vi "Intake Get.vi"(6 "Operator Intake In":T3, 8 "Gripper":bool, 9 "Gripper In":bool, 10 "error in (no error)":errorcluster, 11 "Arm State":bool) -> (0 "error out":errorcluster, 1 "Operator Intake Out":T3)   [LabVIEW 2013]
uses:
  <vilib>/Rock Robotics/WPI/Relay/WPI_RelayValue.ctl
  <vilib>/Rock Robotics/WPI/Solenoid/WPI_SolenoidValue.ctl
panel:
  # "0 < Gripper - Intake\n0 = Gripper - stop\n0 > Gripper - Eject"
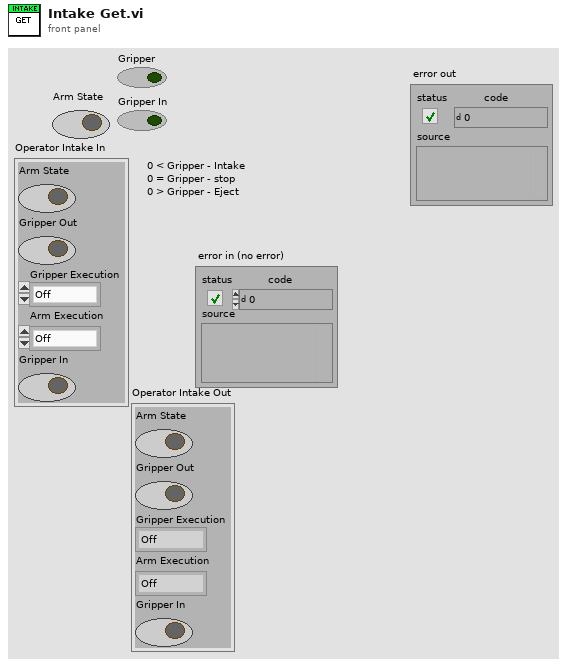
[diagram p1: front panel]
types:
  T1 = typedef "WPI_RelayValue.ctl" = enum16{"Off", "On", "Forward", "Reverse"}
  T2 = typedef "WPI_SolenoidValue.ctl" = enum16{"Off", "On", "Forward", "Reverse"}
  T3 = cluster{"Arm State":bool, "Gripper Out":bool, "Gripper Execution":T1, "Arm Execution":T2, "Gripper In":bool}
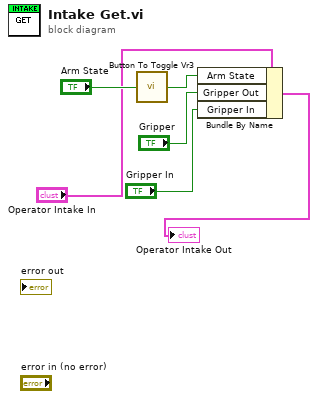
[diagram p0: block diagram]
diagram:
  n1 = call "Button To Toggle Vr3.vi"("InValue"="Arm State") -> ("Result"=w3:bool)
  n2 = Bundle By Name(cluster="Operator Intake In", "Arm State"=w3, "Gripper Out"="Gripper", "Gripper In"="Gripper In") -> (→"Operator Intake Out":T3)
